vi "Midbrain.vi"() -> ()   [LabVIEW 2011]
uses:
  <vilib>/NXT/NXT Controls/ConnectionType.ctl
panel:
  out "Sumo Eyes Raw":i32
  out "IR Seeker Raw":dbl[](array[numeric])
  out "stop 2":bool
  in  "Procedure":i8 min=0 max=7 step=1
  out "Rudder PWM":dbl
  out "Propeller PWM":dbl
  in  "Gain":dbl=0.75
  in  "Distance Setpoiunt":i32=16
  in  "Propeller Speed":i16(slide) scale=-5.0..5.0
  in  "Rudder Pos":i32(slide) scale=-5.0..5.0
  in  "Use XBOX":bool
  out "GoHome":dbl[](array[numeric])
  out "ActCommands":dbl[][](graph)
  out "ActCommand":cluster{"Rudder":i32, "Propeller":i32}
  in  "Debug":bool
  out "AvoidWallCommand":dbl[](array[numeric])
  out "NXTCommand":string
  out "ObsAvoidCommand":dbl[](array[numeric])
  out "SeekIRCommand":dbl[](array[numeric])
  out "PushHomeCommand":dbl[](array[numeric])
  out "WallFollowCommand":dbl[](array[numeric])
  out "Hindbrain Senses":string
  out "Sumo Eyes":i32
  out "Distance Sensor (in)":i32
  out "IR Seeker":i32
  in  "Connection type":T1
  in  "NXT name":string="Sasha Al"
  out "Is Paired with NXT?":bool
  in  "stop":bool
  # "NXT Connection"
  # "Debug"
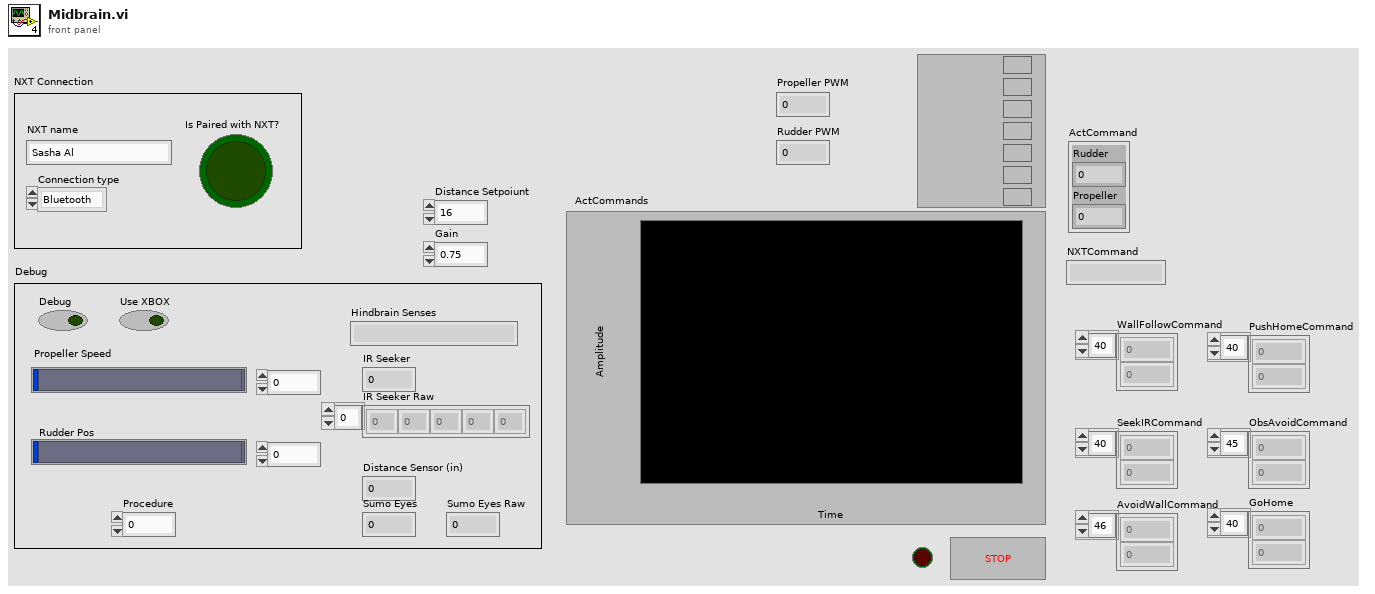
[diagram p1: front panel]
types:
  T1 = typedef "ConnectionType.ctl" = enum16{"Bluetooth", "USB", "WiFi"}
  T2 = typedef "nxt.ctl" = cluster{"nxtHandle":u32, "fileHandle":u32, "fileIterHandle":u32, "moduleHandle":u32, "modIterHandle":u32, "nxtIterHandle":u32}
  T3 = typedef "MidbrainBehaviour.ctl" = cluster{"P-WallFollow":bool, "AvoidWall":bool, "Seek IR":bool, " Push Home":bool, "Go Home":bool}
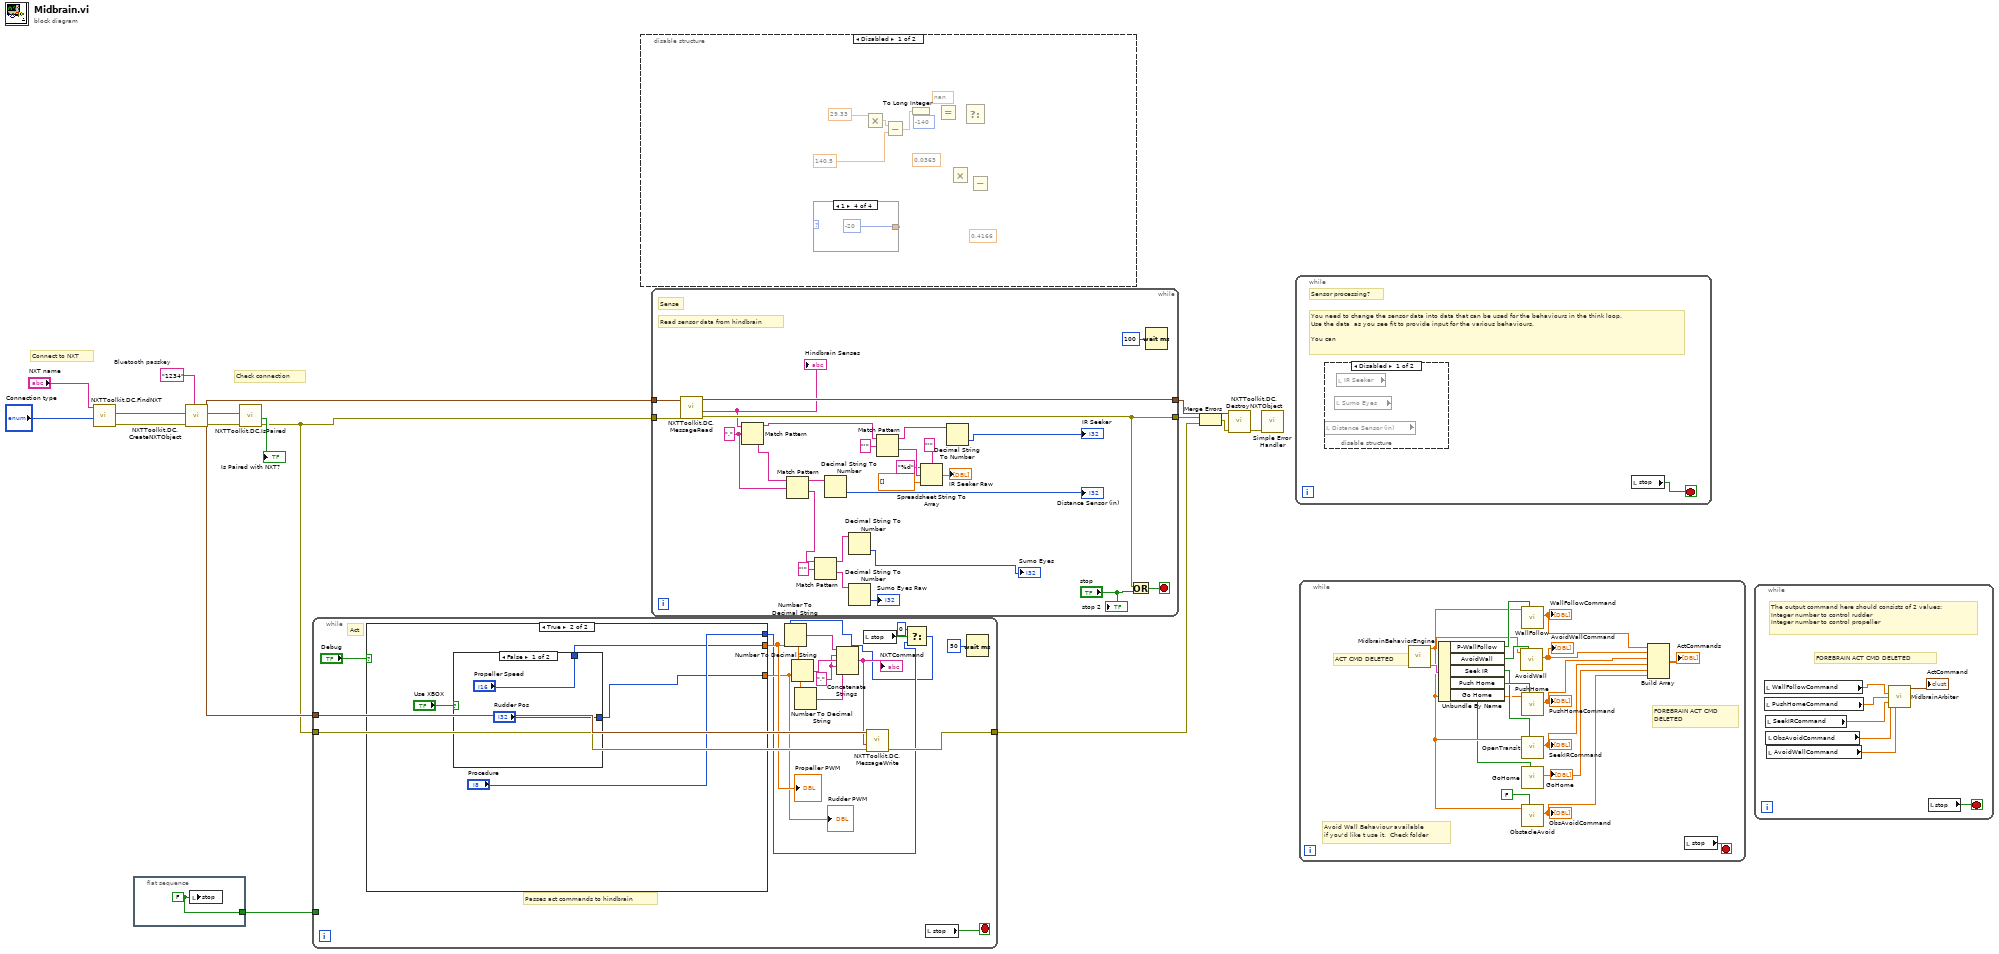
[diagram p0: block diagram]
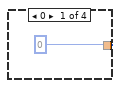
[diagram p2: hidden frame]
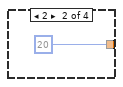
[diagram p3: hidden frame]
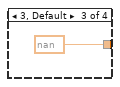
[diagram p4: hidden frame]
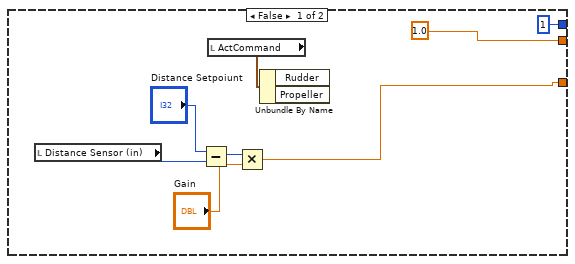
[diagram p7: hidden frame]
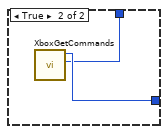
[diagram p8: hidden frame]
diagram:
  w14 = "1234"  # Bluetooth passkey
  # "Check connection"
  # "Connect to NXT"
  n1 = call <vilib>:"NXTToolkit.DC.FindNXT.vi"("Connection type (USB)"="Connection type", "NXT name"="NXT name") -> ("error out"=w13:errorcluster, "VISA resource string"=w12:string)  [unwired: 7 in, 1 out]
  n2 = flat-sequence {
    tunnel: [w17] -> w1
    frame #0 {
      w17 = FALSE ("stop")
      n3 = local write "stop"(w17) -> ()
    }
  }
  n4 = call <vilib>:"NXTToolkit.DC.CreateNXTObject.vi"("Bluetooth passkey (1234)"=w14, "error in (no error)"=w13, "VISA resource string (\"\" : find USB brick)"=w12) -> ("error out"=w11:errorcluster, "VISA resource string out"=w10:string, "NXTObject"=w6:T2)  [unwired: 6 in]
  n5 = call <vilib>:"NXTToolkit.DC.IsPaired.vi"("error in (no error)"=w11, "VISA resource string"=w10) -> ("error out"=w5:errorcluster, "Is Paired?"=→"Is Paired with NXT?":bool)  [unwired: 7 in, 1 out]
  n6 = while {
    tunnel: w6 -> [w34]
    tunnel: w5 -> [w33]
    tunnel: [w32] -> w2
    tunnel: w1 -> [_]
    stop <- w31 stop-if-true
    w22 = "," ("string")
    # "Passes act commands to hindbrain"
    # "Act"
    n7 = case shown="True" "Debug" {
      tunnel: [1.0 ("Propeller Command -5 to 5") w44] -> w25
      tunnel: [w35 w43] -> w24
      tunnel: [i8 1 ("Procedure") "Procedure"] -> w21
      frame False {
        n8 = local read "Distance Sensor (in)"() -> (w41:i32)
        n9 = Subtract(x="Distance Setpoiunt", y=w41) -> (x-y=w39:i32)
        n10 = local read "ActCommand"() -> (w42:cluster{"Rudder":i32, "Propeller":i32})
        n11 = Multiply(x=w39, y="Gain") -> (x*y=w35:dbl)
        n12 = Unbundle By Name(w42) -> ()  [unwired: 2 out]
      }
      frame True {
        n13 = case shown="False" "Use XBOX" {
          tunnel: ["Propeller Speed" w49] -> w44
          tunnel: ["Rudder Pos" w50] -> w43
          frame False {
          }
          frame True {
            n14 = call "XboxGetCommands.vi"() -> ("Prop Command"=w49:i32, "Rudder Command"=w50:i32)  [unwired: 2 in, 2 out]
          }
        }
      }
    }
    "Propeller PWM" <- w25
    "Rudder PWM" <- w24
    n15 = Number To Decimal String(number=w25) -> (decimal integer string=w30:string)  [unwired: 1 in]
    n16 = Number To Decimal String(number=w24) -> (decimal integer string=w29:string)  [unwired: 1 in]
    n17 = local read "stop"() -> (w19:bool)
    n18 = Select(t=i8 0, s=w19, f=w21) -> (s? t:f=w18:i8)
    n19 = Number To Decimal String(number=w18) -> (decimal integer string=w23:string)  [unwired: 1 in]
    n20 = Concatenate Strings(w23, w22, w30, w22, w29) -> (w28:string)
    "NXTCommand" <- w28
    n21 = call <vilib>:"NXTToolkit.DC.MessageWrite.vi"("error in (no error)"=w33, "Message"=w28, "NXTObject"=w34) -> ("error out"=w32:errorcluster)  [unwired: 5 in, 3 out]
    n22 = local read "stop"() -> (w31:bool)
    n23 = Wait (ms)(milliseconds to wait=u32 50) -> ()  [unwired: 1 out]
  }
  n24 = disable-structure shown="Disabled" {
    frame Disabled {
      (unwired) nan ("t")
      (unwired) -140 ("y")
      (unwired) 0.4166
      (unwired) 0.0363
      n25 = case shown="1" w52 {
        tunnel: [0 20 nan -20] -> w51
        frame 0 {
        }
        frame 2 {
        }
        frame 3, Default {
        }
        frame 1 {
        }
      }
      n26 = Multiply(x=29.33) -> (y=w55:dbl, x*y=w56:dbl)
      n27 = Subtract(x=w56, y=140.5) -> (x-y=w53:dbl)
      n28 = To Long Integer(number=w53) -> ()  [unwired: 1 out]
      n29 = Equal?() -> ()  [unwired: 2 in, 1 out]
      n30 = Multiply() -> ()  [unwired: 2 in, 1 out]
      n31 = Select() -> ()  [unwired: 3 in, 1 out]
      n32 = Subtract() -> ()  [unwired: 2 in, 1 out]
    }
    frame Enabled {
    }
  }
  n33 = while {
    tunnel: w5 -> [w84]
    tunnel: [w82] -> w3
    tunnel: w6 -> [w85]
    tunnel: [w83] -> w15
    stop <- w86 stop-if-true
    w80 = "," ("regular expression")
    # "Read sensor data from hindbrain"
    # "Sense"
    n34 = call <vilib>:"NXTToolkit.DC.MessageRead.vi"("error in (no error)"=w84, "NXTObject"=w85) -> ("error out"=w82:errorcluster, "Message"=w73:string, "NXTObject dup"=w83:T2)  [unwired: 4 in, 3 out]
    "Hindbrain Senses" <- w73
    n35 = Match Pattern(string=w73, regular expression=w80) -> (before substring=w78:string, after substring=w81:string)  [unwired: 1 in, 2 out]
    n36 = Match Pattern(string=w81, regular expression=w80) -> (before substring=w79:string, after substring=w66:string)  [unwired: 1 in, 2 out]
    n37 = Match Pattern(string=w66, regular expression="'") -> (before substring=w63:string, after substring=w64:string)  [unwired: 1 in, 2 out]
    n38 = Decimal String To Number(string=w79) -> (number=→"Distance Sensor (in)":i32)  [unwired: 2 in, 1 out]
    n39 = Decimal String To Number(string=w63) -> (number=→"Sumo Eyes":i32)  [unwired: 2 in, 1 out]
    n40 = Decimal String To Number(string=w64) -> (number=→"Sumo Eyes Raw":i32)  [unwired: 2 in, 1 out]
    n41 = Match Pattern(string=w78, regular expression="'") -> (before substring=w76:string, after substring=w75:string)  [unwired: 1 in, 2 out]
    n42 = Spreadsheet String To Array(delimiter (Tab)="'", format string="%d", spreadsheet string=w75, array type (2D Dbl)=dbl[] []) -> (array=→"IR Seeker Raw":dbl[])
    n43 = Decimal String To Number(string=w76) -> (number=→"IR Seeker":i32)  [unwired: 2 in, 1 out]
    n44 = Or(x=w82, y="stop") -> (x .or. y?=w86:bool)
    n45 = Wait (ms)(milliseconds to wait=u32 100) -> ()  [unwired: 1 out]
    "stop 2" <- "stop"
  }
  n46 = Merge Errors(w3, w2) -> (w4:errorcluster)
  n47 = call <vilib>:"NXTToolkit.DC.DestroyNXTObject.vi"("error in (no error)"=w4, "NXTObject"=w15) -> ("error out"=w16:errorcluster)  [unwired: 9 in]
  n48 = call <vilib>:"Simple Error Handler.vi"("error in (no error)"=w16) -> ()  [unwired: 4 in, 5 out]
  n49 = while {
    stop <- w89 stop-if-true
    # "You need to change the sensor data into data that can be used for the behaviours in the think loop. \nUse the data  as you see fit to provide input for the various behaviours.\n\nYou can"
    # "Sensor processing?"
    n50 = disable-structure shown="Disabled" {
      frame Disabled {
        n51 = local read "Distance Sensor (in)"() -> ()  [unwired: 1 out]
        n52 = local read "Sumo Eyes"() -> ()  [unwired: 1 out]
        n53 = local read "IR Seeker"() -> ()  [unwired: 1 out]
      }
      frame Enabled {
      }
    }
    n54 = local read "stop"() -> (w89:bool)
  }
  n55 = while {
    stop <- w105 stop-if-true
    # "FOREBRAIN ACT CMD\nDELETED"
    # "ACT CMD DELETED"
    # "Avoid Wall Behaviour available\nif you'd like t use it.  Check folder"
    n56 = call "MidbrainBehaviorEngine.vi"() -> ("Cluster"=w104:T3, "VelCom"=w98:dbl)  [unwired: 10 in]
    n57 = Unbundle By Name(w104) -> ("P-WallFollow"=w103:bool, "AvoidWall"=w102:bool, "Seek IR"=w99:bool, "Push Home"=w100:bool, "Go Home"=w92:bool)
    n58 = call "AvoidWall.vi"("Inhibit"=w102, "Velocity"=w98) -> ("ActCommand"=w96:dbl[])  [unwired: 7 in, 2 out]
    "AvoidWallCommand" <- w96
    n59 = call "WallFollow.vi"("Inhibit"=w103, "Velocity"=w98) -> ("ActCommand"=w97:dbl[])  [unwired: 7 in, 2 out]
    "WallFollowCommand" <- w97
    n60 = call "PushHome.vi"("Inhibit"=w100, "Velocity"=w98) -> ("ActCommand"=w95:dbl[])  [unwired: 7 in, 2 out]
    "PushHomeCommand" <- w95
    n61 = call "OpenTransit.vi"("Inhibit"=w99, "Velocity"=w98) -> ("ActCommand"=w94:dbl[])  [unwired: 7 in, 2 out]
    "SeekIRCommand" <- w94
    n62 = call "ObstacleAvoid.vi"("Inhibit"=FALSE, "VelCom"=w98) -> ("ActCommand"=w91:dbl[])  [unwired: 8 in, 1 out]
    "ObsAvoidCommand" <- w91
    n63 = call "GoHome.vi"("Inhibit"=w92) -> ("ActCommand"=w90:dbl[])  [unwired: 8 in, 2 out]
    "GoHome" <- w90
    n64 = Build Array(w97, w96, w95, w94, w90, w91) -> (→"ActCommands":dbl[][])
    n65 = local read "stop"() -> (w105:bool)
  }
  n66 = while {
    stop <- w112 stop-if-true
    # "FOREBRAIN ACT CMD DELETED"
    # "The output command here should consists of 2 values:\nInteger number to control rudder\nInteger number to control propeller"
    n67 = local read "WallFollowCommand"() -> (w110:dbl[])
    n68 = local read "PushHomeCommand"() -> (w109:dbl[])
    n69 = local read "SeekIRCommand"() -> (w107:dbl[])
    n70 = local read "ObsAvoidCommand"() -> (w106:dbl[])
    n71 = local read "AvoidWallCommand"() -> (w108:dbl[])
    n72 = call "MidbrainArbiter.vi"("P-WallFollow"=w110, "PushHome"=w109, "SeekIR"=w107, "ObsAvoid"=w106, "AvoidWall"=w108) -> ("ActCommand"=→"ActCommand":cluster{"Rudder":i32, "Propeller":i32})  [unwired: 10 in]
    n73 = local read "stop"() -> (w112:bool)
  }
